vi "Actor Core.vi"(8 "error in":errorcluster, 11 "ServiceManager-DebugView in":refnum<class "ServiceManager-DebugView.lvclass">) -> (0 "error out":errorcluster, 3 "Actor out":refnum<class "Actor.lvclass">)   [LabVIEW 2020, in "ServiceManager-DebugView.lvlib" / "ServiceManager-DebugView.lvclass"]
doc: "(<B>Filename</B>: Actor Framework.lvlib:Actor.lvclass:Actor Core.vi)\n\nReceives messages to the actor, reacts to them, and initiates any error handling that may shut the actor down.\n\nDescendant classes may override this VI to append parallel tasks for the actor to complete while it handles messages. Overrides use the Call Parent Class Method node."
uses:
  ServiceManager-DebugView.lvclass
  <vilib>/ActorFramework/Actor/Actor.lvclass
panel:
  out "String":string
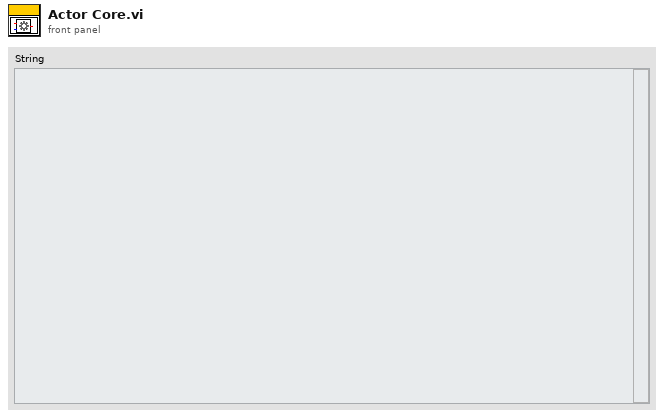
[diagram p1: front panel]
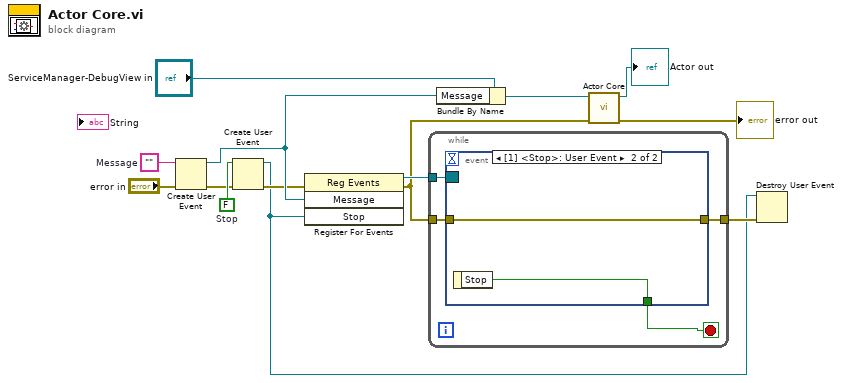
[diagram p0: block diagram]
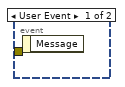
[diagram p2: hidden frame]
diagram:
  w6 = FALSE  # Stop
  w10 = ""  # Message
  n1 = Create User Event(user event datatype=w10, error in="error in") -> (user event=w8:refnum<user-event>, error out=w5:errorcluster)
  n2 = Create User Event(user event datatype=w6, error in=w5) -> (user event=w1:refnum<user-event>, error out=w4:errorcluster)
  n3 = register-events(error in=w4, w8, w1) -> (reference out=w11:refnum<event-registration>, error out=w2:errorcluster)  [unwired: 1 in]
  n4 = while {
    tunnel: w11 -> [w18]
    tunnel: [w16] -> w3
    tunnel: w2 -> [w15]
    stop <- w17 stop-if-true
    n5 = event shown="[1] <Stop>: User Event" {
      selector: w18 -> [_ _]
      dyn-events: _ -> [_ _]
      timeout: _ -> [_ _]
      tunnel: [_ w20] -> w17
      tunnel: [_ w19] -> w16
      tunnel: w15 -> [_ w19]
      event User Event {
        n6 = event-data() -> ()  [unwired: 1 in, 1 out]
      }
      event User Event {
        n7 = event-data() -> ("Stop"=w20:bool)  [unwired: 1 in]
      }
    }
  }
  n8 = Bundle By Name(cluster="ServiceManager-DebugView in", "Message"=w8) -> (w9:refnum<class "ServiceManager-DebugView.lvclass">)
  n9 = call-parent "Actor Core.vi"("error in"=w2, "Actor in"=w9) -> ("error out"=→"error out":errorcluster, "Actor out"=→"Actor out":refnum<class "Actor.lvclass">)  [unwired: 8 in]
  n10 = Destroy User Event(user event=w1, error in=w3) -> ()  [unwired: 1 out]
